vi "Init.vi"() -> (0 "Error Out":errorcluster, 3 "LINX Resource":T1)   [LabVIEW 2016]
uses:
  <vilib>/MakerHub/LINX/Private/Type Defs/Peripherals/SPI/SPI Configuration.ctl
  <vilib>/MakerHub/LINX/Private/Type Defs/Peripherals/SPI/SPI Bit Order.ctl
  <vilib>/MakerHub/LINX/Private/Type Defs/Peripherals/SPI/SPI Mode.ctl
  <vilib>/MakerHub/LINX/Private/Type Defs/LINX Ref.ctl
  <vilib>/MakerHub/LINX/Private/Type Defs/Platform.ctl
  <vilib>/MakerHub/LINX/Private/Type Defs/Interface.ctl
  <vilib>/MakerHub/LINX/Private/Device/Type Defs/LINX Device Config.ctl
  <vilib>/MakerHub/LINX/Private/Device/Type Defs/TCP Config.ctl
  <vilib>/MakerHub/LINX/Private/Device/Type Defs/Channels.ctl
  <vilib>/MakerHub/LINX/Public/Utilities/Open Serial.vi
  <vilib>/MakerHub/LINX/LMH-LINX.lvlib
  <vilib>/MakerHub/LINX/Private/Device/Device.lvlib
panel:
  in  "Serial Port":refnum<visa-resource-name>="COM4"
  out "Actual Clock Frequency":u32
  in  "SPI Configuration":T7={"Clock Frequency"=1000000, "Bit Order"=enum."MSb First", "SPI Mode"=enum."Mode 1"}
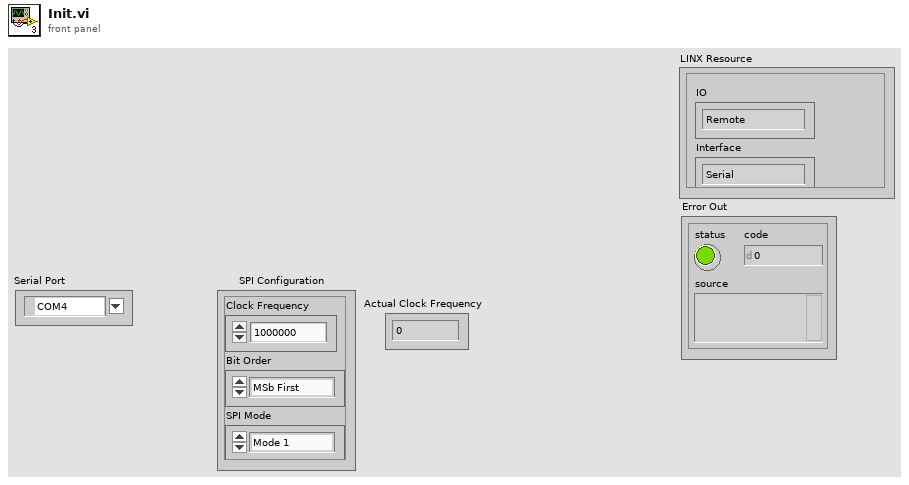
[diagram p1: front panel]
types:
  T1 = typedef "LMH-LINX.lvlib/LINX Ref.ctl" = cluster{"IO":T2, "Interface":T3, "LINX Device Config":T4}
  T2 = typedef "LMH-LINX.lvlib/Platform.ctl" = enum16{"Remote", "Local"}
  T3 = typedef "LMH-LINX.lvlib/Interface.ctl" = enum16{"Serial", "TCP"}
  T4 = typedef "LMH-LINX.lvlib/Device.lvlib/LINX Device Config.ctl" = cluster{"Interface":T3, "COM Port":refnum<visa-resource-name>, "TCP Configuration":T5, "Device Family":u8, "Device ID":u8, "Device Name":string, "TCP Ref":refnum<k5>, "Channels":T6}
  T5 = typedef "LMH-LINX.lvlib/Device.lvlib/TCP Config.ctl" = cluster{"IP Address":string, "Port":u16}
  T6 = typedef "LMH-LINX.lvlib/Channels.ctl" = cluster{"DI":u8[], "DO":u8[], "AI":u8[], "AO":u8[], "PWM":u8[], "QE":u8[], "UART":u8[], "I2C 2":u8[], "SPI":u8[], "CAN":u8[], "Servo":u8[], "AI Ref (V)":dbl, "AI Resolution (Bits)":u8, "AO Ref (V)":dbl, "AO Resolution (Bits)":u8}
  T7 = typedef "LMH-LINX.lvlib/SPI Configuration.ctl" = cluster{"Clock Frequency":u32, "Bit Order":T8, "SPI Mode":T9}
  T8 = typedef "LMH-LINX.lvlib/SPI Bit Order.ctl" = enum8{"LSb First", "MSb First"}
  T9 = typedef "LMH-LINX.lvlib/SPI Mode.ctl" = enum8{"Mode 0", "Mode 1", "Mode 2", "Mode 3"}
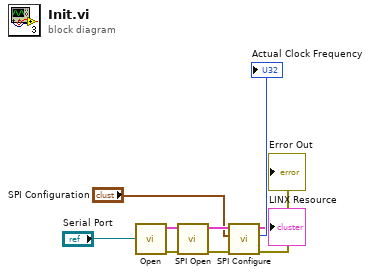
[diagram p0: block diagram]
diagram:
  n1 = call-poly <vilib>:"Open.vi"("Serial Port"="Serial Port") -> ("Error Out"=w6:errorcluster, "LINX Resource"=w9:T1)  [unwired: 8 in, 1 out]
  n2 = call <vilib>:"SPI Open.vi"("Error In"=w6, "LINX Resource"=w9) -> ("Error Out"=w7:errorcluster, "LINX Resource"=w8:T1)  [unwired: 8 in]
  n3 = call <vilib>:"SPI Configure.vi"("Error In"=w7, "SPI Configuration"="SPI Configuration", "LINX Resource"=w8) -> ("Error Out"=→"Error Out":errorcluster, "Actual Clock Frequency"=→"Actual Clock Frequency":u32, "LINX Resource"=→"LINX Resource":T1)  [unwired: 6 in]
